vi "SV Read Newest Data.vi"(7 "reader ID":string="NewestData", 8 "error in (no error)":errorcluster, 9 "timeout (0 ms)":i32, 10 "block length (-1 = all)":i32=-1, 11 "buffer":refnum<data-value>) -> (0 "error out":errorcluster, 1 "end of buffer":bool, 2 "waveforms subset":waveform(dbl)[](array[waveform]), 3 "buffer out":refnum<data-value>)   [LabVIEW 2017]
doc: "Adds buffering to stimulus-response applications. You must manually select the polymorphic instance to use."
uses:
  <vilib>/addons/_NISVFA/_Shared subVIs/Data Objects/Waveforms (DBL)/Waveforms (N Ch).lvclass
  C:/Program Files (x86)/National Instruments/LabVIEW 2017/vi.lib/addons/_NISVFA/_Shared subVIs/Data Objects/Data/Data.lvclass
  <vilib>/addons/_NISVFA/_Shared subVIs/Data Objects/Data/Data.lvclass/Data.ctl
  <vilib>/addons/_NISVFA/_Shared subVIs/Data Objects/Waveforms (DBL)/Waveforms (N Ch).lvclass/Waveforms (N Ch).ctl
  <vilib>/addons/_NISVFA/_Shared subVIs/Data Objects/Waveforms (DBL)/Read Mode for Deleting Stale Data.vi
  <vilib>/addons/_NISVFA/_Shared subVIs/Common/sv_Convert Timestamp to Relative Index.vi
  <vilib>/addons/_NISVFA/_Shared subVIs/Common/SV Get Data Subset.vi
  <vilib>/addons/_NISVFA/_Shared subVIs/Common/svc_Copy Waveform Subset (Index).vi
  <vilib>/addons/_NISVFA/_Shared subVIs/Common/sv_Get NI Property Name String.vi
  <vilib>/addons/_NISVFA/_Shared subVIs/Data Objects/subVIs/Get Oldest of ReaderTimestamps.vi
  <vilib>/addons/_NISVFA/_Shared subVIs/Data Objects/subVIs/Set Data Timestamp.vi
  <vilib>/addons/_NISVFA/_Shared subVIs/Data Objects/subVIs/Set Data Length.vi
  <vilib>/addons/_NISVFA/_Shared subVIs/Common/svc_Get Waveform Subset (Index).vi
  <vilib>/addons/_NISVFA/_Shared subVIs/Common/svc_Copy Array Subset (Index).vi
  <vilib>/addons/_NISVFA/_Shared subVIs/Common/svc_Get Array Subset (Index).vi
  <vilib>/addons/_NISVFA/_Shared subVIs/Common/svc_Coerce Index and Length.vi
  <vilib>/Utility/error.llb/Error Cluster From Error Code.vi
  <vilib>/Utility/error.llb/Trim Whitespace.vi
  <vilib>/ErrorRing/Error Ring.xnode
  <vilib>/addons/_NISVFA/_Shared subVIs/Data Objects/Data/Data.lvclass
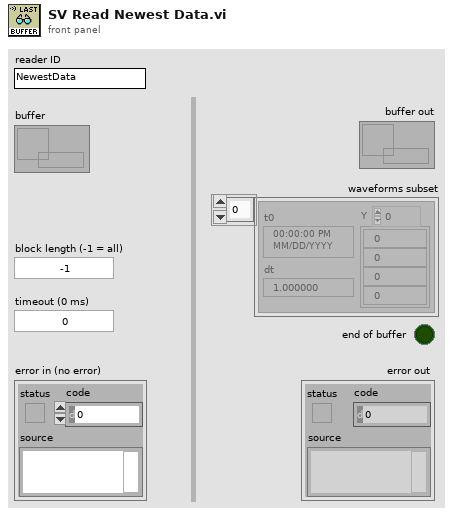
[diagram p1: front panel]
types:
  T1 = enum16{"Data Ready", "First Sample Not Yet Available", "Last Sample Not Yet Available", "Data No Longer Available"}
  T2 = typedef "svc_Delete Data Options (enum).ctl" = enum16{"Write", "Read", "Release"}
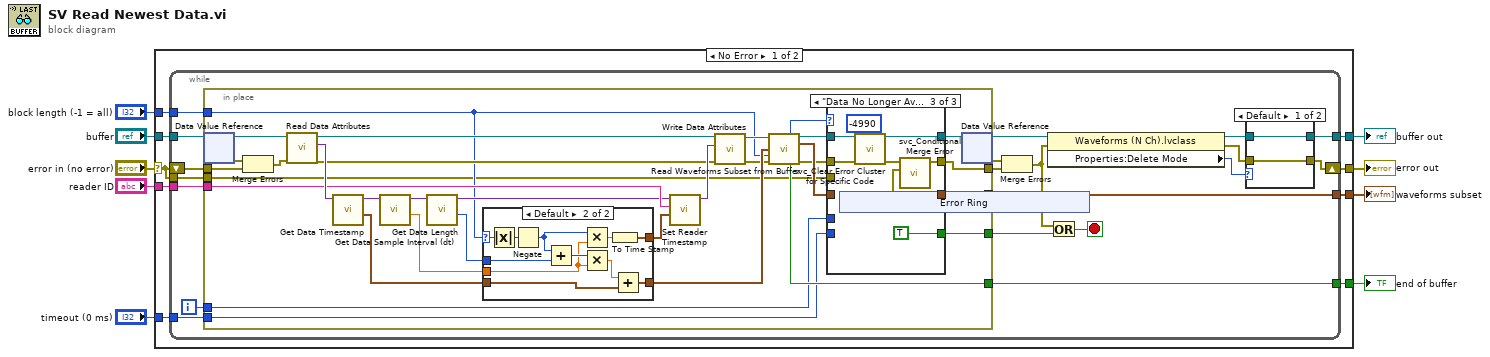
[diagram p0: block diagram]
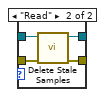
[diagram p2: hidden frame]
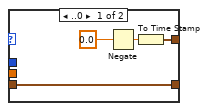
[diagram p3: hidden frame]
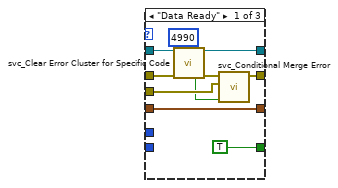
[diagram p4: hidden frame]
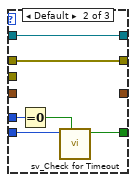
[diagram p5: hidden frame]
diagram:
  n1 = case shown="No Error" "error in (no error)" {
    selector: "error in (no error)" -> [w10 w118]
    tunnel: [w13 w119] -> w9
    tunnel: [w12 w118] -> w8
    tunnel: [w18 _] -> w7
    tunnel: "buffer" -> [w14 w119]
    tunnel: [w17 _] -> w5
    tunnel: "block length (-1 = all)" -> [w16 _]
    tunnel: "reader ID" -> [w15 _]
    tunnel: "timeout (0 ms)" -> [w11 _]
    frame No Error {
      n2 = while {
        tunnel: [w38] -> w18
        tunnel: [w37] -> w17
        tunnel: w16 -> [w36]
        tunnel: w15 -> [w35]
        tunnel: w14 -> [w34]
        tunnel: [w24] -> w13
        shift-right: [w23] -> w12
        shift-left: w10 -> [w33]
        tunnel: w11 -> [w30]
        tunnel: w10 -> [w19]
        i -> [w29]
        stop <- w21 stop-if-true
        n3 = in-place {
          in-place-border: [w76] -> w31
          in-place-border: [w75] -> w38
          in-place-border: [w72] -> w37
          in-place-border: w33 -> [w54]
          in-place-border: w36 -> [w47]
          in-place-border: w35 -> [w61]
          in-place-border: w30 -> [w50]
          in-place-border: w29 -> [w49]
          in-place-border: [w48] -> w20
          in-place-border: w19 -> [w45]
          n4 = in-place-dvr #1(w34) -> (w52:refnum<class "Waveforms (N Ch).lvclass">, w55:errorcluster)
          n5 = Merge Errors(w55, w54) -> (w53:errorcluster)
          n6 = call <vilib>:"Read Data Attributes.vi"("error in (no error)"=w53, "Data in"=w52) -> ("error out"=w58:errorcluster, "data attributes"=w69:variant, "Data out"=w59:refnum<class "Waveforms (N Ch).lvclass">)  [unwired: 7 in]
          n7 = call <vilib>:"Get Data Timestamp.vi"("variant in"=w69) -> ("timestamp"=w65:timestamp, "variant out"=w68:variant)  [unwired: 9 in]
          n8 = call <vilib>:"Get Data Sample Interval (dt).vi"("variant in"=w68) -> ("dt [s]"=w66:dbl, "variant out"=w67:variant)  [unwired: 9 in]
          n9 = call <vilib>:"Get Data Length.vi"("variant in"=w67) -> ("number of samples"=w63:i32, "variant out"=w60:variant)  [unwired: 9 in]
          n10 = case shown="Default" w47 {
            selector: w47 -> [_ w88]
            tunnel: w66 -> [_ w84]
            tunnel: w63 -> [_ w91]
            tunnel: w65 -> [w80 w89]
            tunnel: [w80 w87] -> w64
            tunnel: [w77 w81] -> w46
            frame ..0 {
              n11 = Negate(x=0.0) -> (-x=w78:dbl)
              n12 = To Time Stamp(1:w78) -> (0:w77:timestamp)
            }
            frame Default {
              n13 = Absolute Value(x=w88) -> (abs(x)=w83:i32)
              n14 = Negate(x=w83) -> (-x=w85:i32)
              n15 = Add(x=w85, y=w91) -> (x+y=w90:i32)
              n16 = Multiply(x=w85, y=w84) -> (x*y=w82:dbl)
              n17 = Multiply(x=w90, y=w84) -> (x*y=w86:dbl)
              n18 = To Time Stamp(1:w82) -> (0:w81:timestamp)
              n19 = Add(x=w86, y=w89) -> (x+y=w87:timestamp)
            }
          }
          n20 = call <vilib>:"Set Reader Timestamp.vi"("timestamp"=w46, "ID"=w61, "data attributes in"=w60) -> ("data attributes out"=w62:variant)  [unwired: 8 in]
          n21 = call <vilib>:"Write Data Attributes.vi"("error in (no error)"=w58, "data attributes"=w62, "Data in"=w59) -> ("error out"=w56:errorcluster, "Data out"=w57:refnum<class "Waveforms (N Ch).lvclass">)  [unwired: 7 in]
          n22 = call <vilib>:"Read Waveforms Subset from Buffer.vi"("Waveforms (N Ch)"=w57, "timestamp"=w64, "block length"=w47, "error in (no error)"=w56) -> ("subset status"=w70:T1, "Waveforms (N Ch)"=w74:refnum<class "Waveforms (N Ch).lvclass">, "waveforms subset"=w73:waveform(dbl)[], "end of buffer"=w75:bool, "error out"=w71:errorcluster)  [unwired: 5 in, 2 out]
          n23 = case shown="\"Data No Longer Available\"" w70 {
            tunnel: [w99 w106 w113] -> w51
            tunnel: [w94 w105 w108] -> w76
            tunnel: w74 -> [w99 w106 w113]
            tunnel: w73 -> [w100 _ _]
            tunnel: [w100 _ _] -> w72
            tunnel: w71 -> [w98 w105 w110]
            tunnel: w50 -> [_ w103 _]
            tunnel: w49 -> [_ w102 _]
            tunnel: [TRUE ("timeout") w101 TRUE ("timeout")] -> w48
            tunnel: w45 -> [w95 _ _]
            frame "Data Ready" {
              n24 = call <vilib>:"svc_Clear Error Cluster for Specific Code.vi"("error in (no error)"=w98, "code"=4990) -> ("error cleared"=w92:bool, "error out"=w93:errorcluster)  [unwired: 12 in]
              n25 = call <vilib>:"svc_Conditional Merge Error.vi"("merge"=w92, "new error"=w95, "error in (no error)"=w93) -> ("error out"=w94:errorcluster)  [unwired: 8 in]
            }
            frame Default {
              n26 = Equal To 0?(x=w102) -> (x = 0?=w104:bool)
              n27 = call <vilib>:"sv_Check for Timeout.vi"("reset"=w104, "timeout [ms]"=w103) -> ("timeout"=w101:bool)  [unwired: 8 in, 1 out]
            }
            frame "Data No Longer Available" {
              n28 = xnode "Error Ring"() -> ("error out"=w107:errorcluster)
              n29 = call <vilib>:"svc_Clear Error Cluster for Specific Code.vi"("error in (no error)"=w110, "code"=-4990) -> ("error out"=w109:errorcluster)  [unwired: 12 in, 1 out]
              n30 = call <vilib>:"svc_Conditional Merge Error.vi"("new error"=w107, "error in (no error)"=w109) -> ("error out"=w108:errorcluster)  [unwired: 9 in]
            }
          }
          n31 = in-place-dvr #1(w51) -> (w25:refnum<data-value>, w32:errorcluster)
        }
        n32 = Merge Errors(w32, w31) -> (w22:errorcluster)
        n33 = property class="Waveforms (N Ch).lvclass"(reference=w25, error in=w22) -> (reference out=w27:refnum<data-value>, error out=w26:errorcluster, "Properties:Delete Mode"=w28:T2)
        n34 = Or(x=w22, y=w20) -> (x .or. y?=w21:bool)
        n35 = case shown="Default" w28 {
          tunnel: [w40 w43] -> w24
          tunnel: w27 -> [w40 w44]
          tunnel: w26 -> [w39 w42]
          tunnel: [w39 w41] -> w23
          frame Default {
          }
          frame "Read" {
            n36 = call <vilib>:"Delete Stale Samples.vi"("error in (no error)"=w42, "buffer"=w44) -> ("error out"=w41:errorcluster, "buffer"=w43:refnum<data-value>)  [unwired: 6 in, 2 out]
          }
        }
      }
    }
    frame Error {
    }
  }
  "buffer out" <- w9
  "error out" <- w8
  "waveforms subset" <- w5
  "end of buffer" <- w7
